vi "Read Waveform.vi"(8 "error in (no error)":errorcluster, 10 "Parameters 3":T1={"Source (0: Channel 1)"=0, "Timeout (10000 ms)"=10000} {"Source (0: Channel 1)" items=["Channel 1", "Channel 2", "Channel 3", "Channel 4", "Math", "Reference A", "Reference B", "Reference C", "Reference D", "FFT"]}, 11 "EDUX1002G in":refnum<class "EDUX1002G.lvclass">) -> (0 "error out":errorcluster, 2 "Waveform Data":waveform(dbl)(graph), 3 "EDUX1002G out":refnum<class "EDUX1002G.lvclass">)   [LabVIEW 2020, in "Osciloscope Tektronix.lvlib" / "EDUX1002G.lvclass"]
uses:
  EDUX1002G.lvclass
  C:/Users/Pablo/Osciloscope-Tek/TDS2000/Libraries/Osciloscope Tektronix/Clases/Osciloscope/Osciloscope.lvclass
  Osciloscope/Osciloscope.lvclass/Osciloscope.ctl
  Osciloscope/Read COM.vi
  <instrlib>/Agilent 2000 3000 X-Series/Public/Data/Read Waveforms (Single).vi
  <instrlib>/Agilent 2000 3000 X-Series/Agilent 2000 3000 X-Series.lvlib
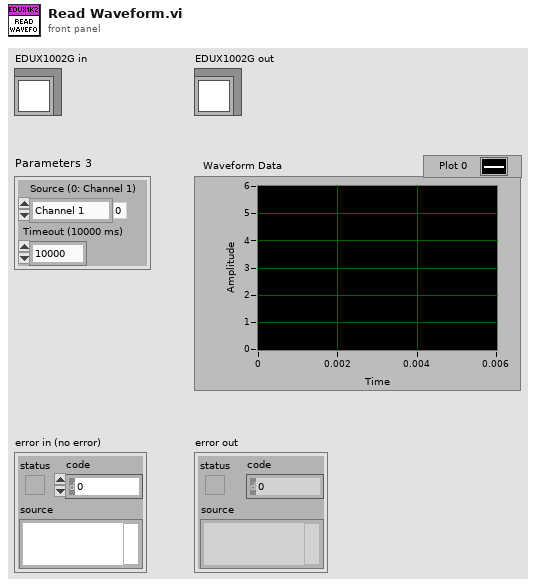
[diagram p1: front panel]
types:
  T1 = cluster{"Source (0: Channel 1)":u16, "Timeout (10000 ms)":u32}
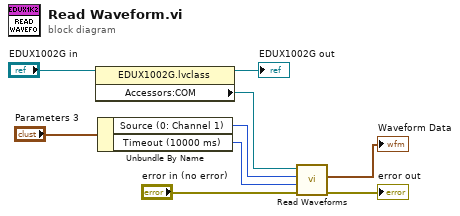
[diagram p0: block diagram]
diagram:
  n1 = property class="EDUX1002G.lvclass"(reference="EDUX1002G in") -> (reference out=→"EDUX1002G out":refnum<class "EDUX1002G.lvclass">, "Accessors:COM"=w5:refnum<visa-resource-name>)  [unwired: 1 in, 1 out]
  n2 = Unbundle By Name("Parameters 3") -> ("Source (0: Channel 1)"=w3:u16, "Timeout (10000 ms)"=w2:u32)
  n3 = call-poly <instrlib>:"Read Waveforms.vi"("error in (no error)"="error in (no error)", "Timeout (10000 ms)"=w2, "Source Channel (0: Channel 1)"=w3, "VISA resource name"=w5) -> ("error out"=→"error out":errorcluster, "Waveform Data"=→"Waveform Data":waveform(dbl))  [unwired: 5 in, 1 out]
